vi "CAN WRITE ONLY.vi"(1 "Extended":bool=TRUE, 2 "Write In":refnum<k21>, 3 "string":string, 4 "ID":string) -> (0 "Write Out":refnum<k21>)   [LabVIEW 2023]
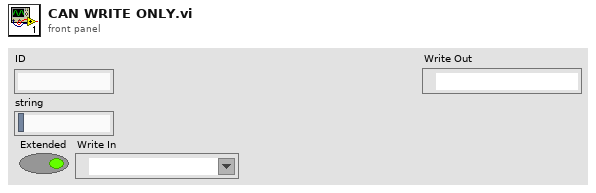
[diagram p1: front panel]
types:
  T1 = typedef "XNET Frame CAN.ctl" = cluster{"timestamp":timestamp, "payload":u8[], "identifier":u32, "type":T2, "extended?":bool, "echo?":bool}
  T2 = typedef "XNET Frame Type CAN.ctl" = u8
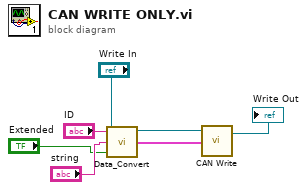
[diagram p0: block diagram]
diagram:
  n1 = call "Data_Convert.vi"("Extended"="Extended", "string"="string", "ID"="ID") -> ("CAN frame"=w6:T1)
  n2 = call "CAN Write.vi"("CAN frame"=w6, "Write In"="Write In") -> ("Write Out"=→"Write Out":refnum<k21>)  [unwired: 1 in, 1 out]
